vi "GettingSerialDataF.vi"() -> ()   [LabVIEW 2020]
uses:
  State2.ctl
  <vilib>/Instr/_visa.llb/VISA Configure Serial Port (Instr).vi
panel:
  in  "VISA resource name (COM)":refnum<visa-resource-name>="CNCB0"
  out "Temperature Graph":T1(graph)
  in  "stop":bool
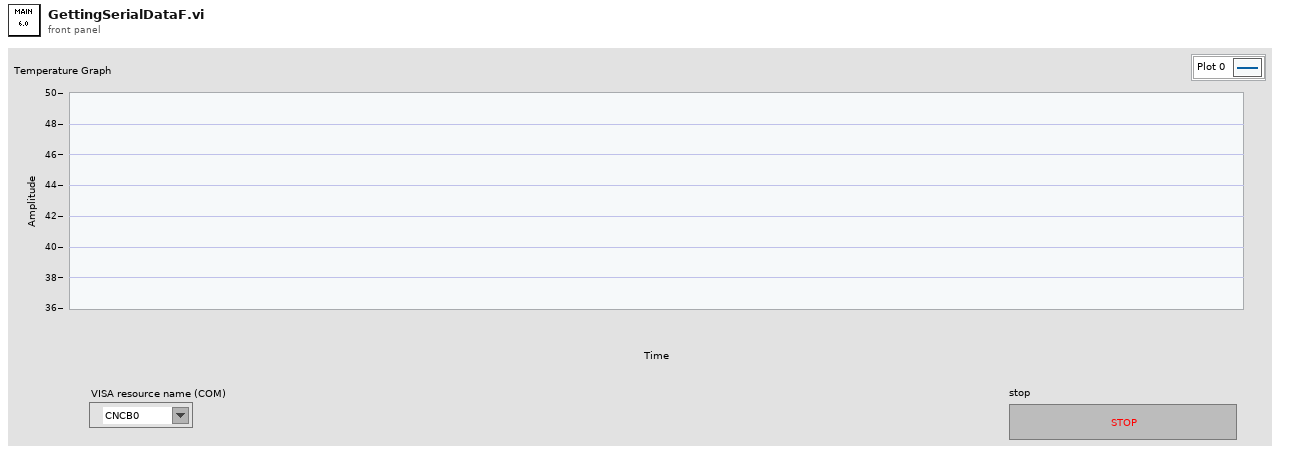
[diagram p1: front panel]
types:
  T1 = cluster{"seconds since 1Jan1904":timestamp, dbl}[]
  T2 = typedef "State2.ctl" = enum16{"Initialize", "ReadSerial", "ShowData", "Finalize"}
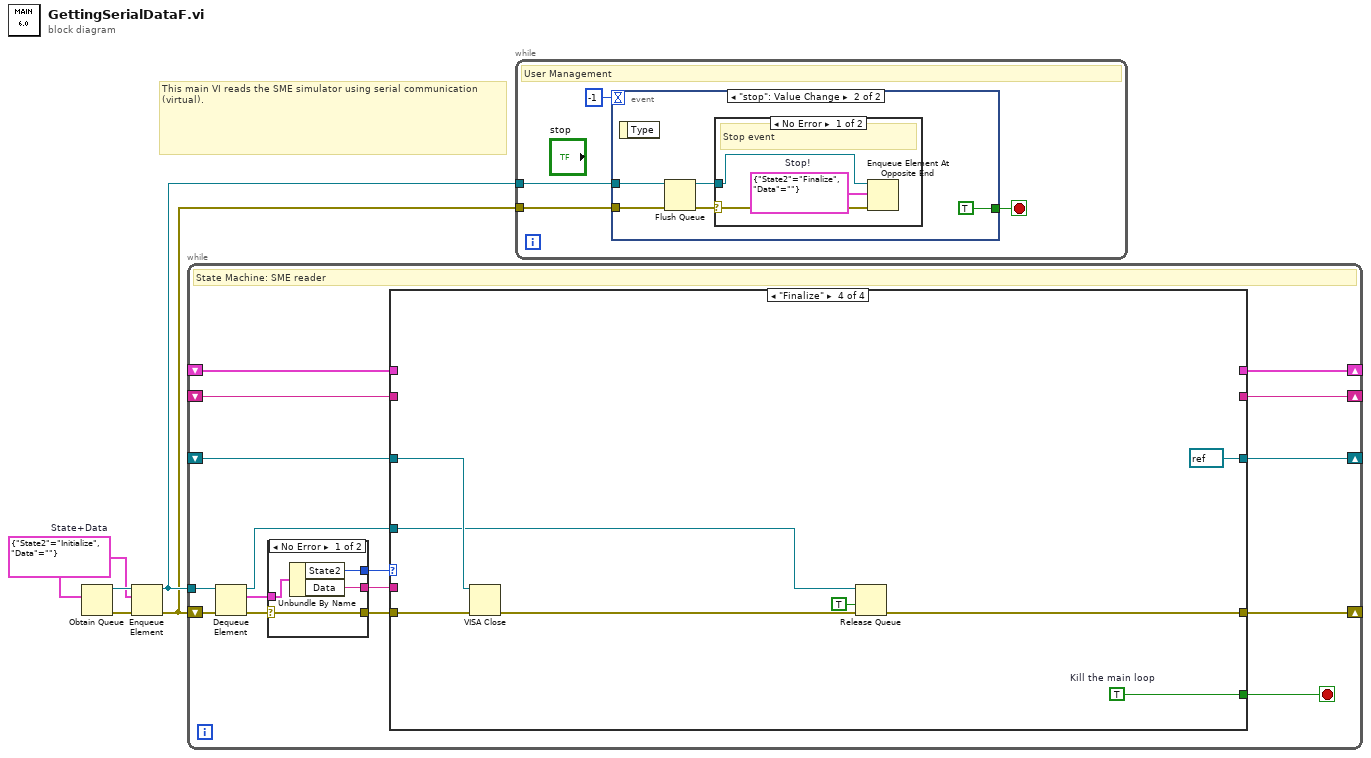
[diagram p0: block diagram]
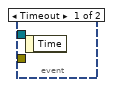
[diagram p2: hidden frame]
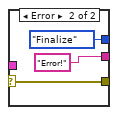
[diagram p4: hidden frame]
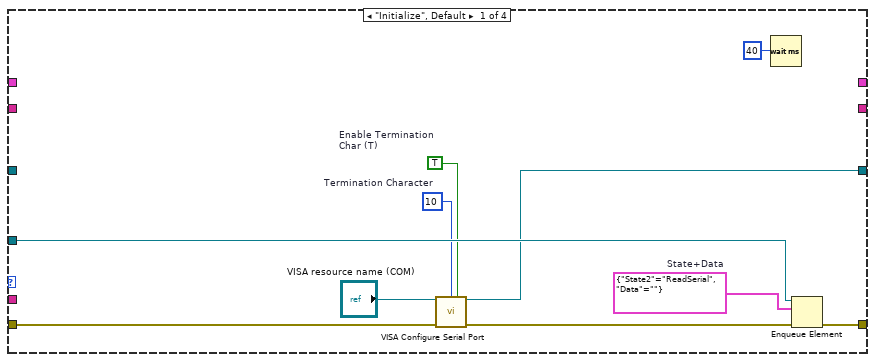
[diagram p5: hidden frame]
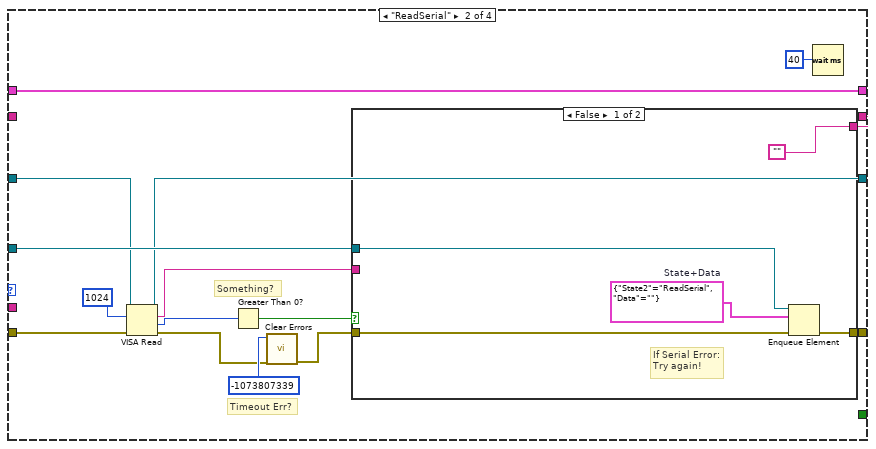
[diagram p6: hidden frame]
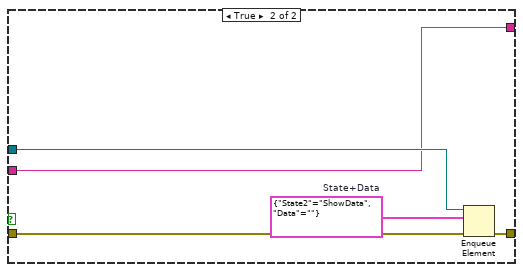
[diagram p7: hidden frame]
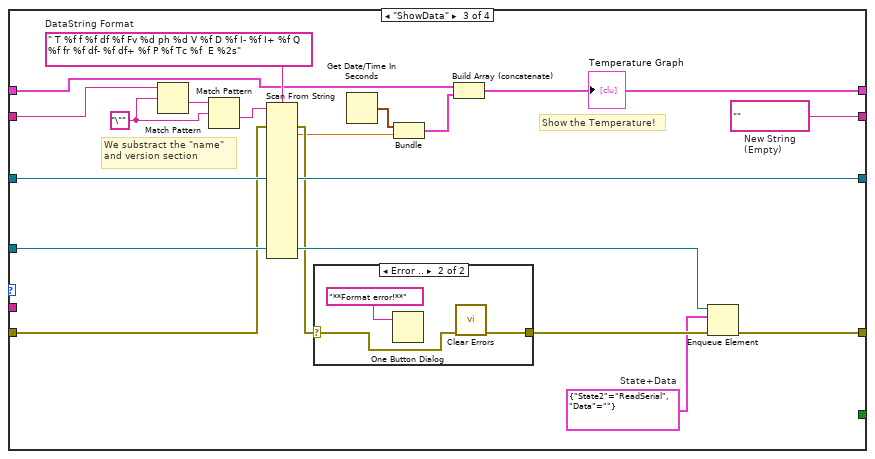
[diagram p8: hidden frame]
diagram:
  w4 = cluster{"State2":T2, "Data":string} {"State2"=enum."Initialize", "Data"=""}  # State+Data
  # "This main VI reads the SME simulator using serial communication (virtual)."
  n1 = Obtain Queue(element data type=w4) -> (queue out=w5:refnum<queue>, error out=w3:errorcluster)  [unwired: 4 in, 1 out]
  n2 = Enqueue Element(queue=w5, element=w4, error in (no error)=w3) -> (queue out=w2:refnum<queue>, error out=w1:errorcluster)  [unwired: 1 in, 1 out]
  n3 = while {
    shift-right: [w18] -> _
    shift-left: w1 -> [w12]
    shift-right: [w17] -> _
    shift-left: _ -> [w16]
    shift-right: [w14] -> _
    shift-left: _ -> [w15]
    tunnel: w2 -> [w13]
    shift-right: [w6] -> _
    shift-left: _ -> [w7]
    stop <- w9 stop-if-true
    # "State Machine: SME reader"
    n4 = Dequeue Element(queue=w13, error in (no error)=w12) -> (queue out=w8:refnum<queue>, element=w10:cluster{"State2":T2, "Data":string}, error out=w11:errorcluster)  [unwired: 1 in, 1 out]
    n5 = case shown="No Error" w11 {
      selector: w11 -> [w22 w27]
      tunnel: w10 -> [w25 _]
      tunnel: [w24 State2."Finalize" ("State2")] -> w21
      tunnel: [w23 "Error!" ("Data")] -> w20
      tunnel: [w22 w27] -> w19
      frame No Error {
        n6 = Unbundle By Name(w25) -> ("State2"=w24:T2, "Data"=w23:string)
      }
      frame Error {
      }
    }
    n7 = case shown="\"Finalize\"" w21 {
      tunnel: w20 -> [_ _ _ _]
      tunnel: w19 -> [w33 w46 w71 w92]
      tunnel: [w37 w52 w78 w89] -> w18
      tunnel: [w32 w44 w81 refnum<visa-resource-name> refnum ("VISA resource name")] -> w17
      tunnel: w16 -> [_ w47 w81 w93]
      tunnel: w15 -> [_ _ w73 _]
      tunnel: [_ w42 w80 _] -> w14
      tunnel: [_ _ _ w90] -> w9
      tunnel: w8 -> [w38 w53 w79 w88]
      tunnel: w7 -> [_ w51 w66 _]
      tunnel: [_ w51 w65 _] -> w6
      frame "Initialize", Default {
        w30 = cluster{"State2":T2, "Data":string} {"State2"=enum."ReadSerial", "Data"=""}  # State+Data
        w35 = u8 10  # Termination Character
        w36 = TRUE  # Enable Termination Char (T)
        n8 = call-poly "VISA Configure Serial Port"("VISA resource name"="VISA resource name (COM)", "termination char\n(0xA = '\\n' = LF)"=w35, "Enable Termination\nChar (T)"=w36, "error in (no error)"=w33) -> ("VISA resource name out"=w32:refnum<visa-resource-name>, "error out"=w31:errorcluster)  [unwired: 10 in]
        n9 = Wait (ms)(milliseconds to wait=u32 40) -> ()  [unwired: 1 out]
        n10 = Enqueue Element(queue=w38, element=w30, error in (no error)=w31) -> (error out=w37:errorcluster)  [unwired: 1 in, 2 out]
      }
      frame "ReadSerial" {
        # "Timeout Err?"
        # "Something?"
        n11 = VISA Read(VISA resource name=w47, byte count=u32 1024, error in (no error)=w46) -> (VISA resource name out=w44:refnum<visa-resource-name>, read buffer=w43:string, return count=w48:u32, error out=w40:errorcluster)
        n12 = Greater Than 0?(x=w48) -> (x > 0?=w45:bool)
        n13 = call <vilib>:"Clear Errors.vi"("error in (no error)"=w40, "specific error code to clear (0: all)"=-1073807339 ("y")) -> ("error out"=w39:errorcluster)  [unwired: 4 in, 1 out]
        n14 = case shown="False" w45 {
          tunnel: w53 -> [w58 w63]
          tunnel: [w57 w62] -> w52
          tunnel: w39 -> [w54 w60]
          tunnel: w43 -> [_ w61]
          tunnel: ["" w61] -> w42
          frame False {
            w55 = cluster{"State2":T2, "Data":string} {"State2"=enum."ReadSerial", "Data"=""}  # State+Data
            # "If Serial Error:\nTry again!"
            n15 = Enqueue Element(queue=w58, element=w55, error in (no error)=w54) -> (error out=w57:errorcluster)  [unwired: 1 in, 2 out]
          }
          frame True {
            w59 = cluster{"State2":T2, "Data":string} {"State2"=enum."ShowData", "Data"=""}  # State+Data
            n16 = Enqueue Element(queue=w63, element=w59, error in (no error)=w60) -> (error out=w62:errorcluster)  [unwired: 1 in, 2 out]
          }
        }
        n17 = Wait (ms)(milliseconds to wait=u32 40) -> ()  [unwired: 1 out]
      }
      frame "ShowData" {
        w64 = cluster{"State2":T2, "Data":string} {"State2"=enum."ReadSerial", "Data"=""}  # State+Data
        w75 = "\"" ("regular expression")
        w72 = " T %f f %f df %f Fv %d ph %d V %f D %f I- %f I+ %f Q %f fr %f df- %f df+ %f P %f Tc %f  E %2s"  # DataString Format
        w80 = ""  # New String (Empty)
        # "We substract the \"name\"\nand version section"
        # "Show the Temperature!"
        n18 = Match Pattern(string=w73, regular expression=w75) -> (after substring=w76:string)  [unwired: 1 in, 3 out]
        n19 = Match Pattern(string=w76, regular expression=w75) -> (after substring=w74:string)  [unwired: 1 in, 3 out]
        n20 = Scan From String(format string=w72, input string=w74, error in=w71) -> (error out=w70:errorcluster, output 1=w68:dbl)  [unwired: 32 in, 2 out]
        n21 = case shown="Error .." w70 {
          selector: w70 -> [w82 w84]
          tunnel: [w82 w83] -> w77
          frame No Error {
          }
          frame Error {
            n22 = One Button Dialog(message="**Format error!**") -> ()  [unwired: 1 in, 1 out]
            n23 = call <vilib>:"Clear Errors.vi"("error in (no error)"=w84) -> ("error out"=w83:errorcluster)  [unwired: 5 in, 1 out]
          }
        }
        n24 = Get Date/Time In Seconds() -> (seconds since 1Jan1904=w69:timestamp)
        n25 = Bundle("seconds since 1Jan1904"=w69, w68) -> (w67:cluster{"seconds since 1Jan1904":timestamp, dbl})  [unwired: 1 in]
        n26 = Build Array (concatenate)(w66, w67) -> (w65:T1)
        "Temperature Graph" <- w65
        n27 = Enqueue Element(queue=w79, element=w64, error in (no error)=w77) -> (error out=w78:errorcluster)  [unwired: 1 in, 2 out]
      }
      frame "Finalize" {
        w90 = TRUE  # Kill the main loop
        n28 = VISA Close(VISA resource name=w93, error in (no error)=w92) -> (error out=w87:errorcluster)
        n29 = Release Queue(queue=w88, force destroy? (F)=TRUE, error in (no error)=w87) -> (error out=w89:errorcluster)  [unwired: 2 out]
      }
    }
  }
  n30 = while {
    tunnel: w2 -> [w95]
    tunnel: w1 -> [w94]
    stop <- w96 stop-if-true
    # "User Management"
    n31 = event shown="[1] \"stop\": Value Change" {
      selector: _ -> [_ _]
      dyn-events: _ -> [_ _]
      timeout: -1 -> [_ _]
      tunnel: [_ TRUE] -> w96
      tunnel: w95 -> [_ w100]
      tunnel: w94 -> [_ w101]
      event Timeout {
        n32 = event-data() -> ()  [unwired: 1 in, 1 out]
      }
      event "stop": Value Change {
        n33 = event-data() -> ()  [unwired: 1 in, 1 out]
        n34 = Flush Queue(queue=w100, error in (no error)=w101) -> (queue out=w99:refnum<queue>, error out=w98:errorcluster)  [unwired: 1 out]
        n35 = case shown="No Error" w98 {
          selector: w98 -> [w104 _]
          tunnel: w99 -> [w105 _]
          frame No Error {
            w103 = cluster{"State2":T2, "Data":string} {"State2"=enum."Finalize", "Data"=""}  # Stop!
            # "Stop event"
            n36 = Enqueue Element At Opposite End(queue=w105, element=w103, error in (no error)=w104) -> ()  [unwired: 1 in, 3 out]
          }
          frame Error {
            # "Already dead"
          }
        }
      }
    }
  }
